vi "LJM_eReadAddresses.vi"(0 "Handle In":i32, 1 "NumFrames (Auto-Detect)":i32=-1, 5 "aAddresses":i32[](array[numeric]), 7 "aTypes":i32[](array[numeric]), 11 "error in":errorcluster) -> (4 "Handle Out":i32, 10 "aValues":dbl[](array[numeric]) format="%.2f", 14 "ErrorAddress":i32, 15 "error out":errorcluster)   [LabVIEW 2025]
uses:
  Library/Frameworks/LabJackM.framework
panel:
  # "1/20/2015:  Default value of NumFrames changed to -1 which\nequates to Auto-Detect.  If NumFrames = -1, then the NumFrames\ncontrol is ignored and the size of aNames/aAddresses is used to\ndetermine how many frames there are."
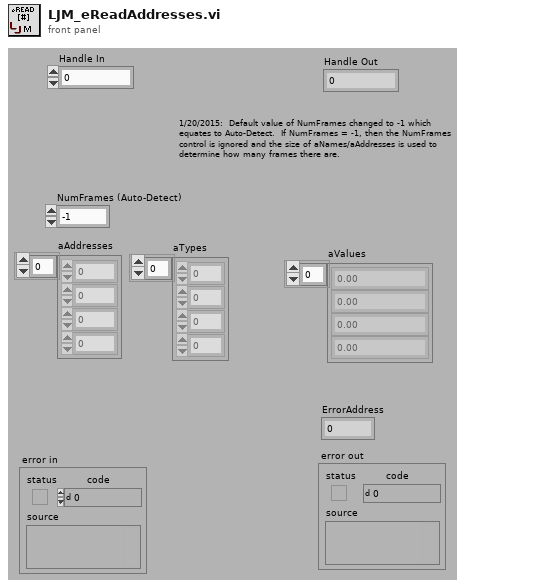
[diagram p1: front panel]
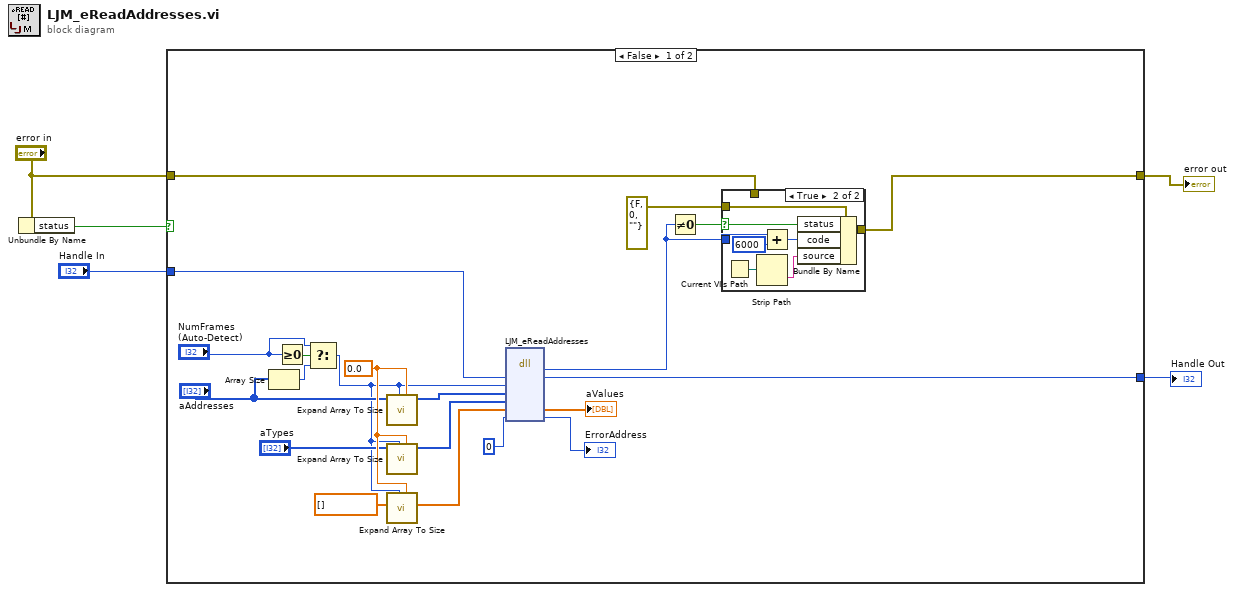
[diagram p0: block diagram]
diagram:
  n1 = Unbundle By Name("error in") -> ("status"=w5:bool)
  n2 = case shown="False" w5 {
    tunnel: "error in" -> [w23 w37]
    tunnel: [w22 w37] -> w3
    tunnel: [w12 w36] -> w2
    tunnel: "Handle In" -> [w11 w36]
    frame False {
      w20 = 0.0 ("Default Value")
      n3 = Array Size(array="aAddresses") -> (size(s)=w10:i32)
      n4 = Greater Or Equal To 0?(x="NumFrames (Auto-Detect)") -> (x >= 0?=w9:bool)
      n5 = Select(t="NumFrames (Auto-Detect)", s=w9, f=w10) -> (s? t:f=w6:i32)
      n6 = call "Expand Array To Size.vi"("Default Value"=w20, "# Elements"=w6, "I32 Array In"="aAddresses") -> ("I32 Array Out"=w21:i32[])  [unwired: 4 in, 4 out]
      n7 = call "Expand Array To Size.vi"("Default Value"=w20, "# Elements"=w6, "I32 Array In"="aTypes") -> ("I32 Array Out"=w18:i32[])  [unwired: 4 in, 4 out]
      n8 = call "Expand Array To Size.vi"("Default Value"=w20, "# Elements"=w6, "DBL Array In"=dbl[] []) -> ("DBL Array Out"=w16:dbl[])  [unwired: 4 in, 4 out]
      n9 = dll-call lib="Library/Frameworks/LabJackM.framework" fn="LJM_eReadAddresses"("Handle"=w11, "NumFrames"=w6, "aAddresses"=w21, "aTypes"=w18, "aValues"=w16, "ErrorFrame"=u32 0) -> ("return type"=w26:i32, "Handle"=w12:i32, "aValues"=→"aValues":dbl[], "ErrorFrame"=→"ErrorAddress":i32)  [unwired: 6 in, 2 out]
      n10 = Not Equal To 0?(x=w26) -> (x != 0?=w25:bool)
      n11 = case shown="True" w25 {
        selector: w25 -> [_ w34]
        tunnel: [w27 w35] -> w22
        tunnel: errorcluster {"status"=FALSE, "code"=0, "source"=""} ("error IO") -> [_ w33]
        tunnel: w26 -> [_ w29]
        tunnel: w23 -> [w27 _]
        frame False {
        }
        frame True {
          n12 = Current VI's Path() -> (path=w31:path)
          n13 = Strip Path(path=w31) -> (name=w32:string)  [unwired: 1 out]
          n14 = Add(x=w29, y=6000) -> (x+y=w30:i32)
          n15 = Bundle By Name(cluster=w33, "status"=w34, "code"=w30, "source"=w32) -> (w35:errorcluster)
        }
      }
    }
    frame True {
    }
  }
  "error out" <- w3
  "Handle Out" <- w2
